vi "Populate Copy.vi"(8 "error in (no error)":errorcluster, 10 "Msg to Populate":refnum<class "Multi Instrument Msg.lvclass">, 11 "Source Msg":refnum<class "Flex Msg.lvclass">) -> (0 "error out":errorcluster, 2 "Populated Msg":refnum<class "Multi Instrument Msg.lvclass">)   [LabVIEW 2020, in "Instrument Handler.lvlib" / "Multi Instrument Msg.lvclass"]
doc: "Populate 'Msg to Populate' with data from 'Source Msg'. Use this VI if some private data is required for the operation of the message and cannot be written in any other way (as in nested message execution).\n\nThis implementation populates the Alias and Core tables with only the required instruments."
uses:
  Multi Instrument Msg.lvclass
  C:/Current projects/WS/PPL/HDH.Actor Framework.Core.Msg.lvlibp/Flex Msg/Flex Msg.lvclass
  PPL/HDH.Actor Framework.Core.Msg.lvlibp/Flex Msg/Flex Msg.lvclass
  PPL/HDH.Actor Framework.Core.Sequencer.lvlibp/Sequencer Core/Sequencer Core.lvclass
  Multi Instrument Msg.lvclass/Multi Instrument Msg.ctl
  Instrument Msg/Instrument Msg.lvclass
  Instrument Handler/Instrument Handler.lvclass
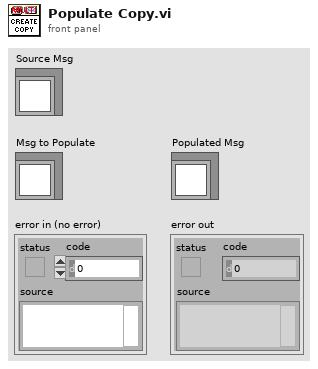
[diagram p1: front panel]
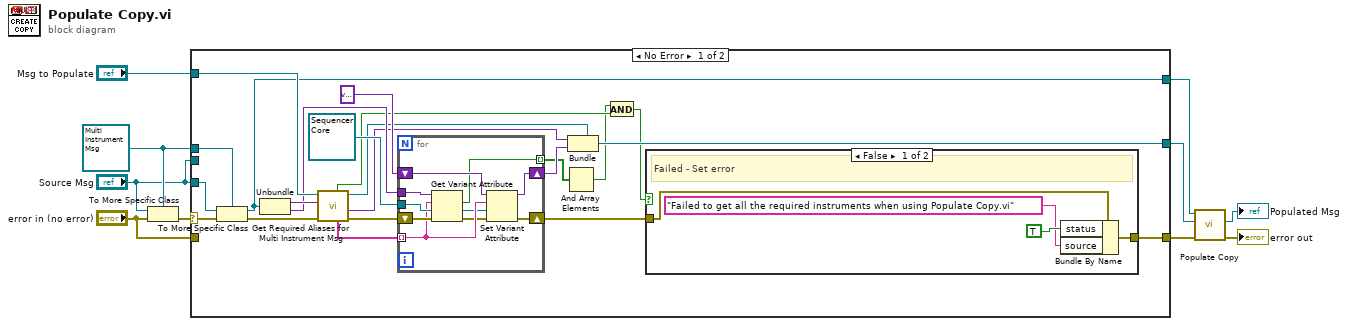
[diagram p0: block diagram]
diagram:
  w4 = refnum<class "Multi Instrument Msg.lvclass"> refnum ("Msg to Populate 2")
  n1 = To More Specific Class(target class=w4, reference="Source Msg", error in="error in (no error)") -> (error out=w8:errorcluster)  [unwired: 1 out]
  n2 = case shown="No Error" w8 {
    selector: w8 -> [w32 _]
    tunnel: [w17 w50] -> w7
    tunnel: "Source Msg" -> [_ w50]
    tunnel: [w12 w49] -> w6
    tunnel: "error in (no error)" -> [_ w49]
    tunnel: w4 -> [w31 _]
    tunnel: "Source Msg" -> [w30 _]
    tunnel: [w18 w48] -> w2
    tunnel: "Msg to Populate" -> [w28 w48]
    frame No Error {
      n3 = To More Specific Class(target class=w31, reference=w30, error in=w32) -> (specific class reference=w17:refnum<class "Multi Instrument Msg.lvclass">, error out=w27:errorcluster)
      n4 = Unbundle(w17) -> (w29:variant, w25:variant)
      n5 = call "Get Required Aliases for Multi Instrument Msg.vi"("error in (no error)"=w27, "Alias Table in"=w29, "Multi Instrument Msg in"=w28) -> ("error out"=w24:errorcluster, "Alias Sub Table"=w20:variant, "Multi Instrument Msg out"=w21:refnum<class "Multi Instrument Msg.lvclass">, "Alias Array"=w26:string[], "All Instruments Present?"=w15:bool)  [unwired: 3 in, 1 out]
      n6 = for {
        tunnel: w26 -> [w44] mode=indexing
        tunnel: w25 -> [w47]
        tunnel: refnum<class "Sequencer Core.lvclass"> refnum ("Owner") -> [w46]
        shift-right: [w42] -> w19
        shift-left: variant -> [w43]
        shift-right: [w39] -> w11
        shift-left: w24 -> [w45]
        tunnel: [w38] -> w16 mode=indexing
        n7 = Get Variant Attribute(Variant=w47, name=w44, default value (empty Variant)=w46, error in=w45) -> (found=w38:bool, value=w40:refnum<class "Sequencer Core.lvclass">, error out=w41:errorcluster)  [unwired: 1 out]
        n8 = Set Variant Attribute(Variant=w43, name=w44, value=w40, error in=w41) -> (Variant out=w42:variant, error out=w39:errorcluster)  [unwired: 1 out]
      }
      n9 = And Array Elements(Boolean array=w16) -> (logical AND=w14:bool)
      n10 = Bundle(cluster=w21, w20, w19) -> (w18:refnum<class "Multi Instrument Msg.lvclass">)
      n11 = And(x=w14, y=w15) -> (x .and. y?=w13:bool)
      n12 = case shown="False" w13 {
        tunnel: [w35 w37] -> w12
        tunnel: w11 -> [w36 w37]
        frame False {
          # "Failed - Set error"
          n13 = Bundle By Name(cluster=w36, "status"=TRUE, "source"="Failed to get all the required instruments when using Populate Copy.vi") -> (w35:errorcluster)
        }
        frame True {
          # "Success"
        }
      }
    }
    frame Error {
    }
  }
  n14 = call-parent "Populate Copy.vi"("error in (no error)"=w6, "Msg to Populate"=w2, "Source Msg"=w7) -> ("error out"=→"error out":errorcluster, "Populated Msg"=→"Populated Msg":refnum<class "Multi Instrument Msg.lvclass">)  [unwired: 7 in]
